vi "Program list Selection_R0.vi"(8 "error in":errorcluster, 9 "FeedBack Channel":string[](array[string])=["fgdgfvcbc", "vnfhgjkn", "21354682"], 10 "Filepath":path=path "D:/My Project/2019-2020/Magnetic Mareli UM/MM_UM/Project Setup/data/program seq/Program_280A.bin", 11 "vi referenceIn":refnum<vi>) -> (0 "error out":errorcluster, 1 "Exit":bool, 2 "String":string, 3 "vi reference Out":refnum<vi>)   [LabVIEW 2015]
uses:
  Control Button/Exit.ctl
  Control Button/next.ctl
  Galobal variable_TI.vi
panel:
  out "String 2":string
  in  "Next":T1
  in  "Exit":T2
  in  "Program List":string(combo)
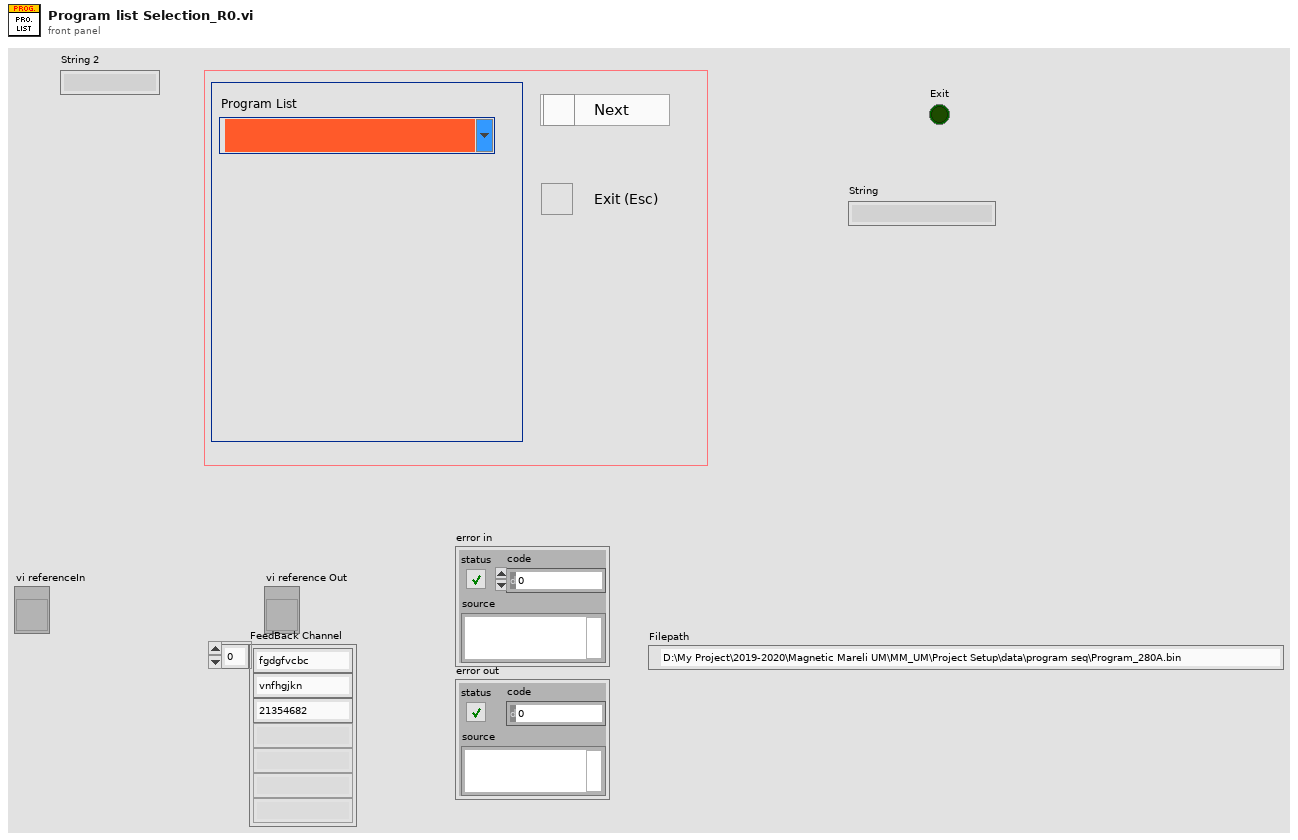
[diagram p1: front panel]
types:
  T1 = typedef "next.ctl" = bool
  T2 = typedef "Exit.ctl" = bool
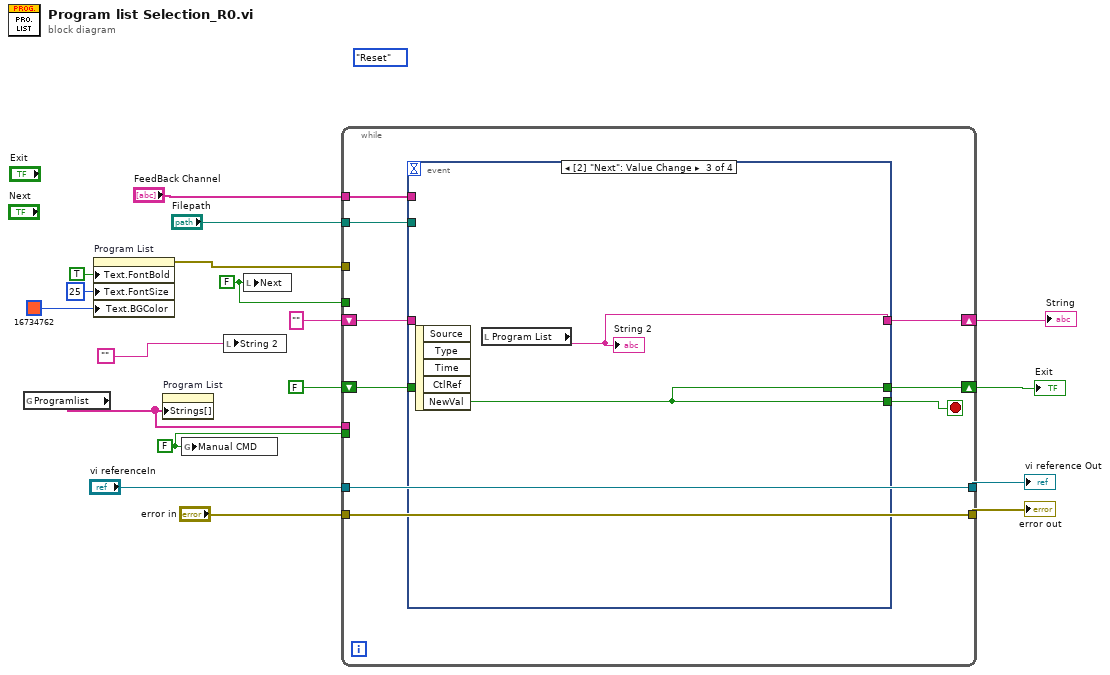
[diagram p0: block diagram]
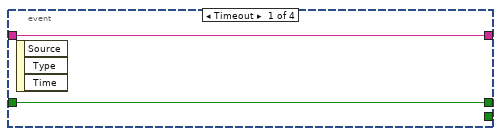
[diagram p2: hidden frame]
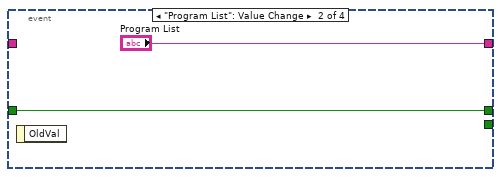
[diagram p3: hidden frame]
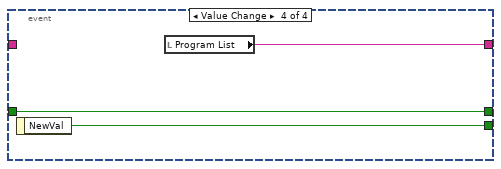
[diagram p4: hidden frame]
diagram:
  (unwired) enum16{"Home", "Reset"}."Reset"
  w7 = FALSE ("Manual CMD")
  w8 = FALSE ("Next")
  n1 = global read "Galobal variable_TI.vi" "Programlist"() -> (w14:string[])
  n2 = property on="Program List" class="CmbBox"("Text.FontBold"=TRUE ("Text.Font:Bold"), "Text.FontSize"=u32 25 ("Text.Font:Size"), "Text.BGColor"=u32 16734762 ("Color Box")) -> (error out=w11:errorcluster)  [unwired: 2 in, 1 out]
  n3 = property on="Program List" class="CmbBox"("Strings[]"=w14) -> ()  [unwired: 2 in, 2 out]
  n4 = global write "Galobal variable_TI.vi" "Manual CMD"(w7) -> ()
  n5 = local write "String 2"("") -> ()
  n6 = local write "Next"(w8) -> ()
  n7 = while {
    shift-right: [w27] -> w18
    shift-left: "" ("Combo Box") -> [w26]
    shift-right: [w24] -> w15
    shift-left: T2 FALSE ("NewVal") -> [w23]
    tunnel: w14 -> [_]
    tunnel: w11 -> [_]
    tunnel: w8 -> [_]
    tunnel: w7 -> [_]
    tunnel: "vi referenceIn" -> [w22]
    tunnel: [w22] -> w5
    tunnel: "error in" -> [w21]
    tunnel: [w21] -> w3
    tunnel: "Filepath" -> [w20]
    tunnel: "FeedBack Channel" -> [w19]
    stop <- w25 stop-if-true
    n8 = event shown="[2] \"Next\": Value Change" {
      selector: _ -> [_ _ _ _]
      dyn-events: _ -> [_ _ _ _]
      timeout: _ -> [_ _ _ _]
      tunnel: [w29 "Program List" w32 w35] -> w27
      tunnel: w26 -> [w29 _ _ _]
      tunnel: [_ _ w33 w36] -> w25
      tunnel: [w28 w30 w33 w34] -> w24
      tunnel: w23 -> [w28 w30 _ w34]
      tunnel: w20 -> [_ _ _ _]
      tunnel: w19 -> [_ _ _ _]
      event Timeout {
        n9 = event-data() -> ()  [unwired: 1 in, 3 out]
      }
      event "Program List": Value Change {
        n10 = event-data() -> ()  [unwired: 1 in, 1 out]
      }
      event Value Change {
        n11 = event-data() -> ("NewVal"=w33:T1)  [unwired: 1 in, 4 out]
        n12 = local read "Program List"() -> (w32:string)
        "String 2" <- w32
      }
      event Value Change {
        n13 = event-data() -> ("NewVal"=w36:T2)  [unwired: 1 in]
        n14 = local read "Program List"() -> (w35:string)
      }
    }
  }
  "String" <- w18
  "Exit" <- w15
  "vi reference Out" <- w5
  "error out" <- w3
